vi "ListTableWHERE.vi"(7 "Jsonconfig":string, 8 "error in (no error)":errorcluster, 10 "condition":string="TEMATY.uruchomienie_tematy_do_uruchomienia", 11 "table":string="TEMATY.uruchomienie_tematy_do_uruchomienia") -> (0 "error out":errorcluster, 3 "data":string[][](array[string]))   [LabVIEW 2017]
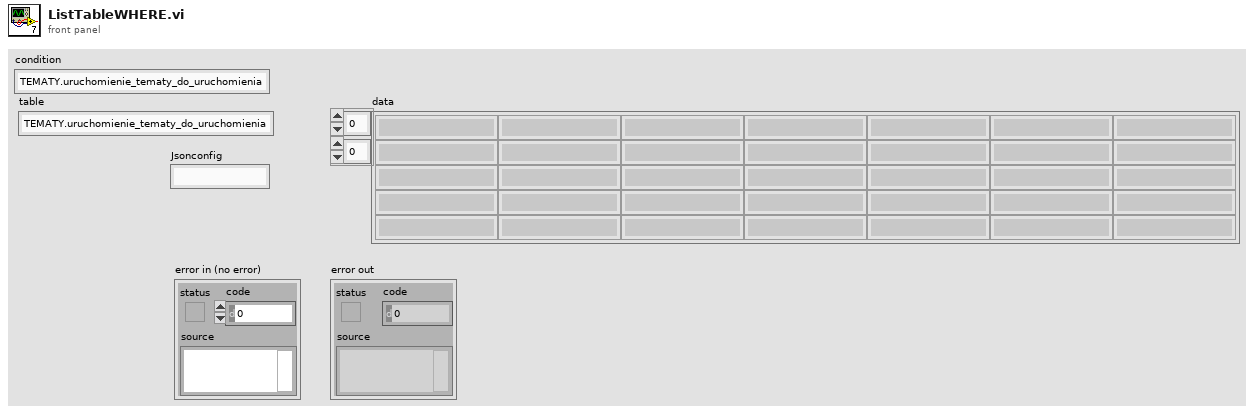
[diagram p1: front panel]
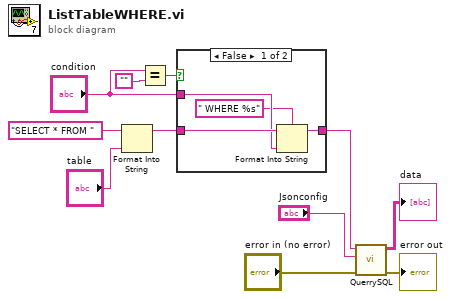
[diagram p0: block diagram]
diagram:
  n1 = Format Into String(initial string="SELECT * FROM ", "table") -> (resulting string=w3:string)  [unwired: 2 in, 1 out]
  n2 = Equal?(x="condition", y="") -> (x = y?=w4:bool)
  n3 = case shown="False" w4 {
    tunnel: [w12 w16] -> w2
    tunnel: w3 -> [w15 w16]
    tunnel: "condition" -> [w14 _]
    frame False {
      n4 = Format Into String(format string=" WHERE %s", initial string=w15, w14) -> (resulting string=w12:string)  [unwired: 1 in, 1 out]
    }
    frame True {
    }
  }
  n5 = call "QuerrySQL.vi"("error in (no error)"="error in (no error)", "Jsonconfig"="Jsonconfig", "String"=w2) -> ("error out"=→"error out":errorcluster, "Array"=→"data":string[][])  [unwired: 7 in]
